vi "Analysis View.vi"(8 "error in (no error)":errorcluster, 11 "Data":T1) -> (0 "error out":errorcluster)   [LabVIEW 2020]
uses:
  Data Cluster.ctl
  Helper Classes/Test Finder/Test Finder.lvclass
panel:
  in  "Method Test Times":i32(listbox)
  out "Histogram":cluster{"X":dbl, "Y":dbl}[](graph)
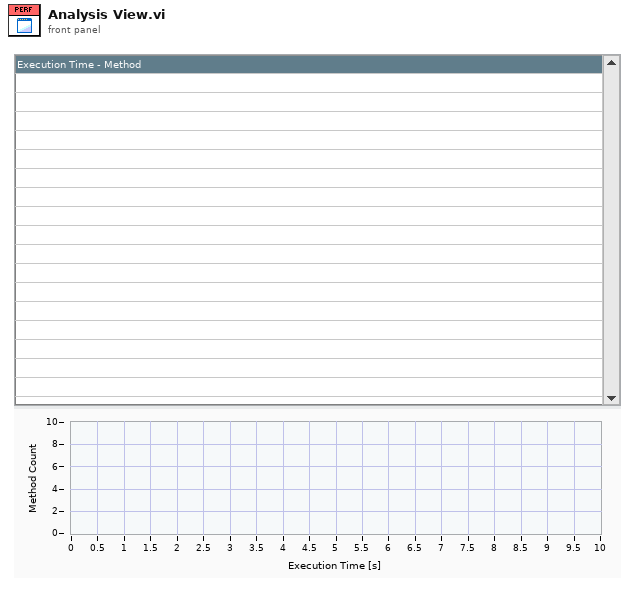
[diagram p1: front panel]
types:
  T1 = typedef "Data Cluster.ctl" = cluster{"Timing Results":map{string, dbl}, "Tags":string[], "Test Finder":refnum<class "Test Finder.lvclass">}
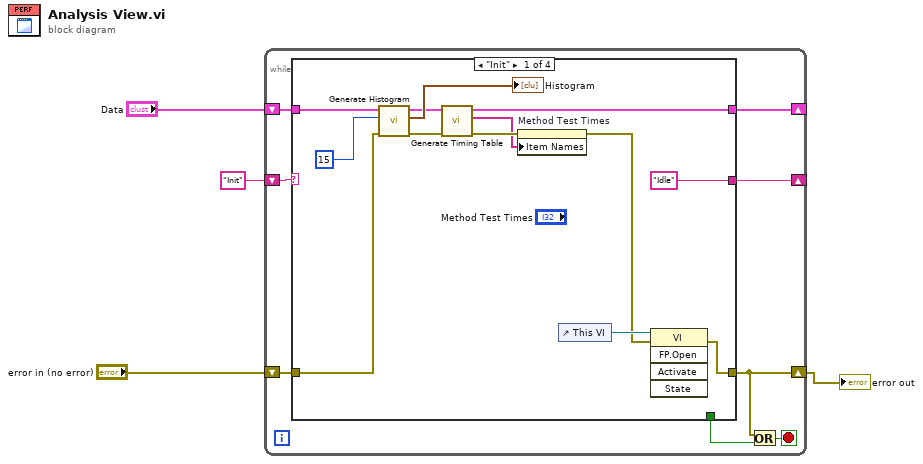
[diagram p0: block diagram]
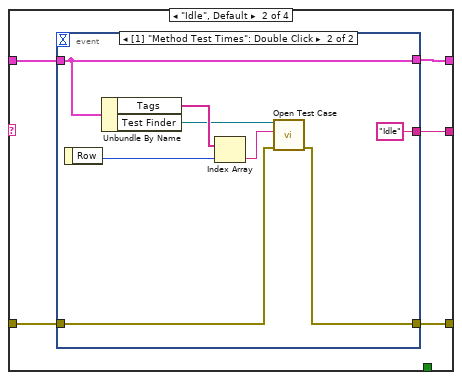
[diagram p2: hidden frame]
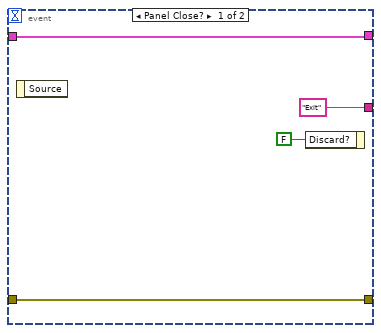
[diagram p3: hidden frame]
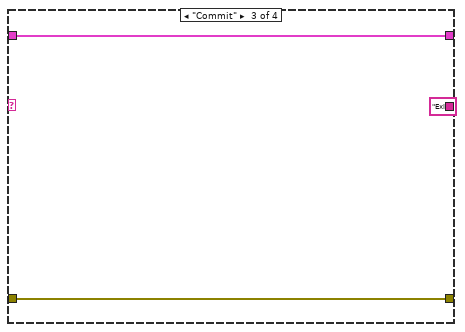
[diagram p4: hidden frame]
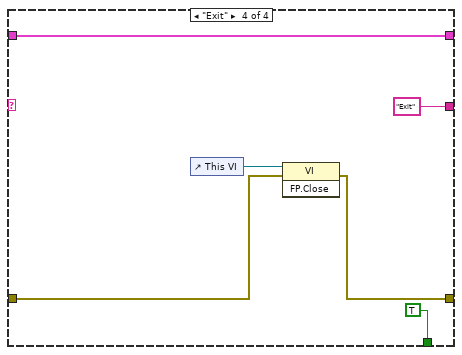
[diagram p5: hidden frame]
diagram:
  n1 = while {
    shift-right: [w9] -> _
    shift-left: "Data" -> [w10]
    shift-right: [w5] -> w2
    shift-left: "error in (no error)" -> [w11]
    shift-right: [w8] -> _
    shift-left: "Init" -> [w12]
    stop <- w6 stop-if-true
    n2 = case shown="\"Init\"" w12 {
      tunnel: [w19 w30 w45 w47] -> w5
      tunnel: w11 -> [w22 w29 w45 w46]
      tunnel: w10 -> [w24 w28 w44 w51]
      tunnel: [w17 w27 w44 w51] -> w9
      tunnel: ["Idle" w26 "Exit" "Exit"] -> w8
      tunnel: [_ _ _ TRUE] -> w7
      frame "Init" {
        n3 = call "Generate Histogram.vi"("error in (no error)"=w22, "Interval Scaling"=u8 15 ("Number of intervals"), "Performance Analyzer In"=w24) -> ("error out"=w16:errorcluster, "Histogram"=→"Histogram":cluster{dbl, dbl}[], "Performance Analyzer Out"=w18:T1)  [unwired: 6 in]
        n4 = call "Generate Timing Table.vi"("error in (no error)"=w16, "Performance Analyzer In"=w18) -> ("error out"=w15:errorcluster, "Timing List"=w13:string[], "Performance Analyzer Out"=w17:T1)  [unwired: 7 in]
        n5 = property on="Method Test Times" class="LstBox (strict)"(error in=w15, "Item Names"=w13) -> (error out=w14:errorcluster)  [unwired: 1 in, 1 out]
        n6 = control-ref of="This VI"() -> (w20:refnum<vi>)
        n7 = invoke class="VI" method="FP.Open"(reference=w20, error in=w14) -> (error out=w19:errorcluster)  [unwired: 3 in, 4 out]
      }
      frame "Idle", Default {
        n8 = event shown="[1] \"Method Test Times\": Double Click" {
          selector: _ -> [_ _]
          dyn-events: _ -> [_ _]
          timeout: _ -> [_ _]
          tunnel: [w34 w36] -> w30
          tunnel: w29 -> [w34 w35]
          tunnel: w28 -> [w33 w42]
          tunnel: [w33 w42] -> w27
          tunnel: ["Exit" "Idle"] -> w26
          event Panel Close? {
            n9 = event-data() -> ()  [unwired: 1 in, 1 out]
            n10 = event-data("Discard?"=FALSE) -> ()  [unwired: 1 in, 1 out]
          }
          event "Method Test Times": Double Click {
            n11 = event-data() -> ("Row"=w40:i32)  [unwired: 1 in]
            n12 = Unbundle By Name(w42) -> ("Tags"=w41:string[], "Test Finder"=w38:refnum<class "Test Finder.lvclass">)
            n13 = Index Array(array=w41, index=w40) -> (element=w37:string)
            n14 = call "Open Test Case.vi"("error in (no error)"=w35, "Tag"=w37, "Test Finder In"=w38) -> ("error out"=w36:errorcluster)  [unwired: 6 in, 2 out]
          }
        }
      }
      frame "Commit" {
      }
      frame "Exit" {
        n15 = control-ref of="This VI"() -> (w48:refnum<vi>)
        n16 = invoke class="VI" method="FP.Close"(reference=w48, error in=w46) -> (error out=w47:errorcluster)  [unwired: 1 in, 2 out]
      }
    }
    n17 = Or(x=w5, y=w7) -> (x .or. y?=w6:bool)
  }
  "error out" <- w2
